vi "hysteresis_PI_with_sat.vi"(4 "wsat_s":sgl[](array[numeric])=[0.0, 0.0, 0.0, 0.0, 0.0, 0.0, 0.0], 5 "N_sat":i32, 6 "d_s":sgl[](array[numeric])=[0.0, 0.0, 0.0, 0.0, 0.0, 0.0, 0.0], 7 "N_hyst":i32, 8 "y_vec_in":sgl[](array[numeric])=[0.0, 0.0, 0.0, 0.0, 0.0, 0.0, 0.0], 9 "w_s":sgl[](array[numeric])=[0.0, 0.0, 0.0, 0.0, 0.0, 0.0, 0.0], 10 "r_s":sgl[](array[numeric])=[0.0, 0.0, 0.0, 0.0, 0.0, 0.0, 0.0], 11 "uk":sgl format="%#_13g") -> (0 "y_vec_out":sgl[](array[numeric]), 3 "H_of_ik":sgl)   [LabVIEW 2017]
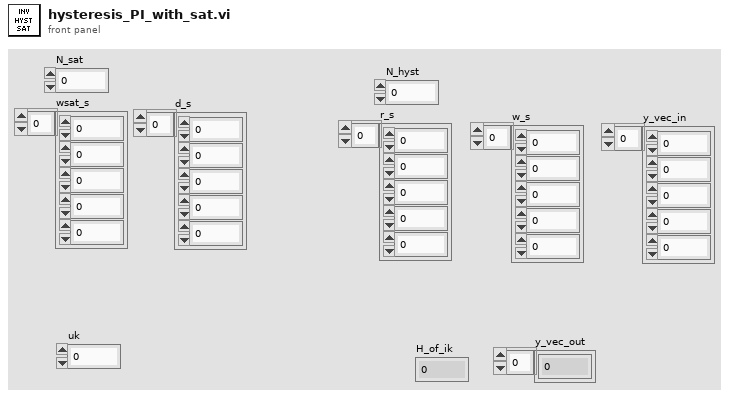
[diagram p1: front panel]
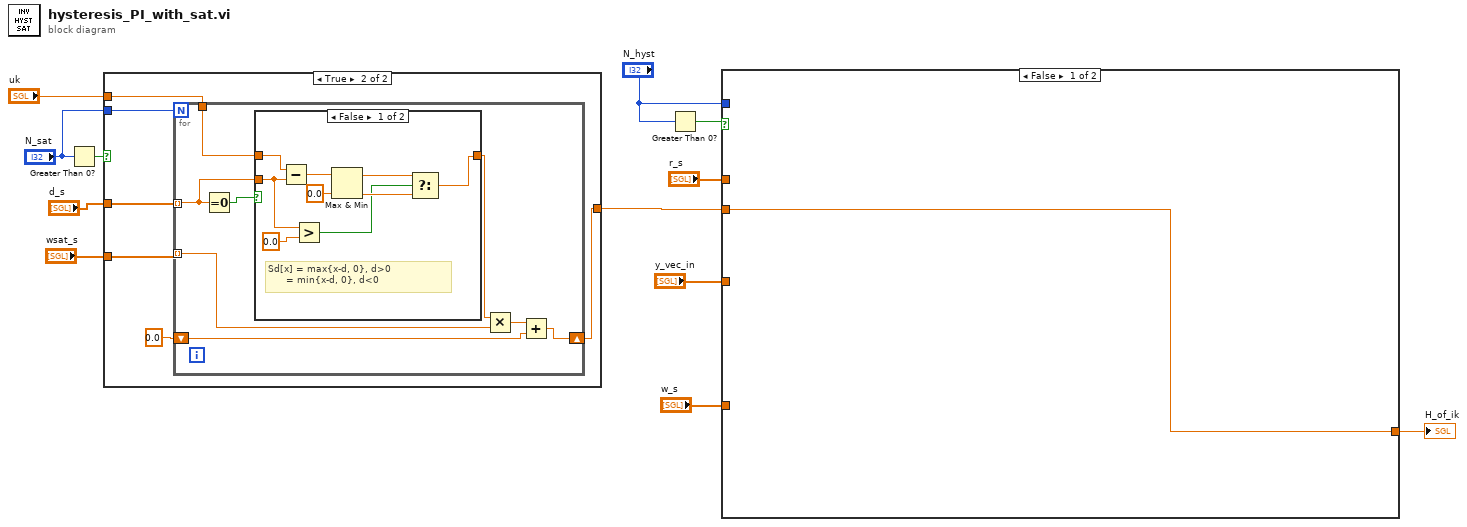
[diagram p0: block diagram]
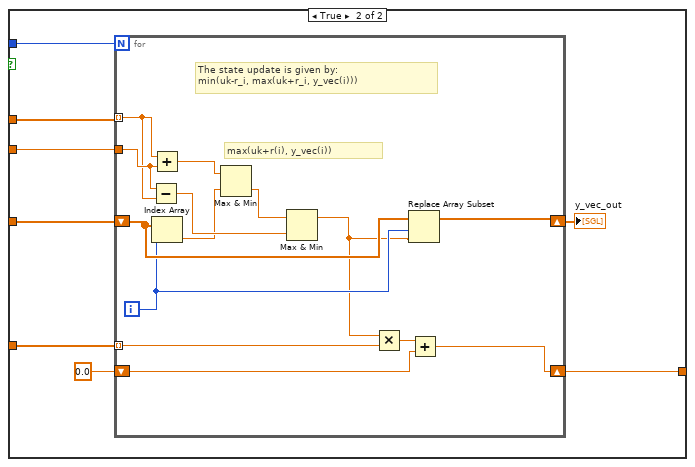
[diagram p4: hidden frame]
diagram:
  n1 = Greater Than 0?(x="N_sat") -> (x > 0?=w9:bool)
  n2 = case shown="True" w9 {
    tunnel: "uk" -> [w13 w18]
    tunnel: "N_sat" -> [_ w19]
    tunnel: [w13 w16] -> w6
    tunnel: "d_s" -> [_ w15]
    tunnel: "wsat_s" -> [_ w14]
    frame False {
    }
    frame True {
      n3 = for {
        N: w19 -> [_]
        tunnel: w18 -> [w26]
        tunnel: w14 -> [w23] mode=indexing
        tunnel: w15 -> [w20] mode=indexing
        shift-right: [w21] -> w16
        shift-left: sgl 0.0 -> [w22]
        n4 = Equal To 0?(x=w20) -> (x = 0?=w27:bool)
        n5 = case shown="False" w27 {
          tunnel: w26 -> [w36 w37]
          tunnel: [w32 w37] -> w24
          tunnel: w20 -> [w29 _]
          frame False {
            # "Sd[x] = max{x-d, 0}, d>0\n      = min{x-d, 0}, d<0"
            n6 = Subtract(x=w36, y=w29) -> (x-y=w35:sgl)
            n7 = Greater?(x=w29, y=sgl 0.0) -> (0:w28:bool)
            n8 = Max & Min(x=w35, y=sgl 0.0) -> (max(x,y)=w33:sgl, min(x,y)=w31:sgl)
            n9 = Select(t=w33, s=w28, f=w31) -> (s? t:f=w32:sgl)
          }
          frame True {
            # "Sd[x] = x, if d = 0"
          }
        }
        n10 = Multiply(x=w24, y=w23) -> (x*y=w25:sgl)
        n11 = Add(x=w25, y=w22) -> (x+y=w21:sgl)
      }
    }
  }
  n12 = Greater Than 0?(x="N_hyst") -> (x > 0?=w11:bool)
  n13 = case shown="False" w11 {
    tunnel: "N_hyst" -> [_ w46]
    tunnel: [w38 w43] -> w12
    tunnel: w6 -> [w38 w42]
    tunnel: "r_s" -> [_ w41]
    tunnel: "y_vec_in" -> [_ w40]
    tunnel: "w_s" -> [_ w39]
    frame False {
    }
    frame True {
      n14 = for {
        N: w46 -> [_]
        tunnel: w39 -> [w54] mode=indexing
        tunnel: w41 -> [w58] mode=indexing
        shift-right: [w51] -> w43
        shift-left: sgl 0.0 -> [w52]
        tunnel: w42 -> [w59]
        shift-right: [w50] -> w44
        shift-left: w40 -> [w49]
        i -> [w48]
        # "max(uk+r(i), y_vec(i))"
        # "The state update is given by:\nmin(uk-r_i, max(uk+r_i, y_vec(i)))"
        n15 = Subtract(x=w59, y=w58) -> (x-y=w56:sgl)
        n16 = Add(x=w58, y=w59) -> (x+y=w60:sgl)
        n17 = Index Array(array=w49, index=w48) -> (element=w55:sgl)
        n18 = Max & Min(x=w60, y=w55) -> (min(x,y)=w57:sgl)  [unwired: 1 out]
        n19 = Max & Min(x=w57, y=w56) -> (max(x,y)=w47:sgl)  [unwired: 1 out]
        n20 = Multiply(x=w47, y=w54) -> (x*y=w53:sgl)
        n21 = Replace Array Subset(array=w49, new element=w47, index=w48) -> (w50:sgl[])
        n22 = Add(x=w53, y=w52) -> (x+y=w51:sgl)
      }
      "y_vec_out" <- w44
    }
  }
  "H_of_ik" <- w12
